vi "rs3_ClampValues.vi"(9 "MinZ":u16=100, 10 "MaxZ":u16=10000, 11 "Depth map":dbl[][](array[numeric])) -> (2 "Array":dbl[][](array[numeric]), 3 "Density (fill factor)":dbl=1.0 format="%_3g")   [LabVIEW 2017, in "libRealSense3.lvlib"]
uses:
  libRealSense3.lvlib
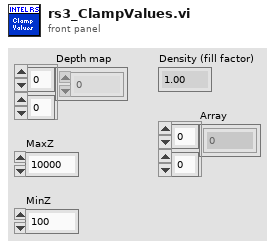
[diagram p1: front panel]
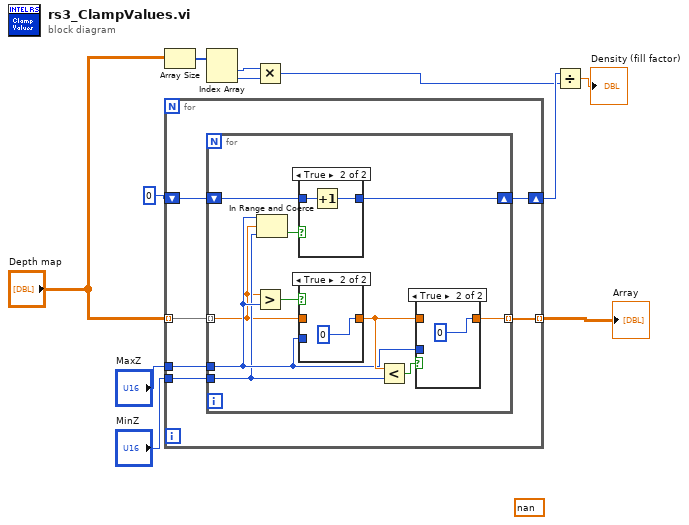
[diagram p0: block diagram]
diagram:
  (unwired) nan ("mean")
  n1 = Array Size(array="Depth map") -> (size(s)=w5:i32[])
  n2 = for {
    tunnel: [w17] -> w10 mode=indexing
    tunnel: "Depth map" -> [w16] mode=indexing
    tunnel: "MaxZ" -> [w15]
    tunnel: "MinZ" -> [w14]
    shift-right: [w12] -> w9
    shift-left: u16 0 -> [w13]
    n3 = for {
      tunnel: [w25] -> w17 mode=indexing
      tunnel: w16 -> [w21] mode=indexing
      tunnel: w15 -> [w23]
      tunnel: w14 -> [w22]
      shift-right: [w18] -> w12
      shift-left: w13 -> [w19]
      n4 = Greater?(x=w21, y=w23) -> (0:w27:bool)
      n5 = In Range and Coerce(upper limit=w23, x=w21, lower limit=w22) -> (In Range?=w20:bool)  [unwired: 1 out]
      n6 = case shown="True" w20 {
        tunnel: w19 -> [w28 w30]
        tunnel: [w28 w29] -> w18
        frame False {
        }
        frame True {
          n7 = Increment(x=w30) -> (x+1=w29:u16)
        }
      }
      n8 = case shown="True" w27 {
        tunnel: w23 -> [_ _]
        tunnel: [w33 u16 0] -> w24
        tunnel: w21 -> [w33 _]
        frame False {
        }
        frame True {
        }
      }
      n9 = Less?(x=w24, y=w22) -> (x < y?=w26:bool)
      n10 = case shown="True" w26 {
        tunnel: w23 -> [_ _]
        tunnel: [w31 u16 0] -> w25
        tunnel: w24 -> [w31 _]
        frame False {
        }
        frame True {
        }
      }
    }
  }
  "Array" <- w10
  n11 = Index Array(array=w5) -> (element #1=w6:i32, element #2=w7:i32)  [unwired: 2 in]
  n12 = Multiply(x=w6, y=w7) -> (x*y=w8:i32)
  n13 = Divide(x=w9, y=w8) -> (x/y=→"Density (fill factor)":dbl)
